vi "SS2 Live_Create HDF5 File Path.vi"(8 "error in (no error)":errorcluster, 9 "File Index":u32, 10 "File Name":string, 11 "File Folder":path) -> (0 "error out":errorcluster, 3 "File path":path)   [LabVIEW 2019]
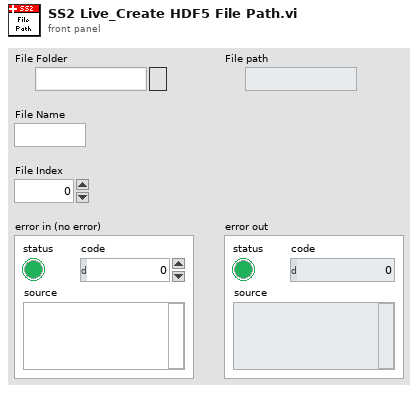
[diagram p1: front panel]
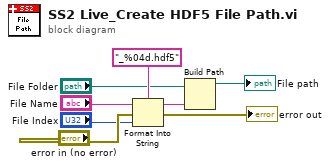
[diagram p0: block diagram]
diagram:
  n1 = Format Into String(format string="_%04d.hdf5", initial string="File Name", error in="error in (no error)", "File Index") -> (resulting string=w5:string, error out=→"error out":errorcluster)
  n2 = Build Path(base path="File Folder", name or relative path=w5) -> (appended path=→"File path":path)
